vi "Init.vi"(8 "error in (no error)":errorcluster, 10 "PictRef":refnum<vi>, 11 "Menu in":refnum<class "Menu.lvclass">) -> (0 "error out":errorcluster, 2 "MenuSelectionEvent":refnum<user-event>, 3 "Menu out":refnum<class "Menu.lvclass">)   [LabVIEW 2021, in "Menu.lvlib" / "Menu.lvclass"]
uses:
  Menu.lvclass
  MenuSelection.ctl
  Data.ctl
  MenuItems.ctl
  <vilib>/Utility/miscctls.llb/LVMenuShortCut.ctl
  Picture2D/src/Picture/Image.lvclass
  TD_CloseEvent.ctl
  MenuColors.ctl
  Picture2D/src/Color/Color.lvclass
  Picture2D/src/Font/Font.lvclass
  SubMenuIcon.ctl
  Picture2D/src/Picture2D/Picture2D.lvclass
  Menu.lvclass/Menu.ctl
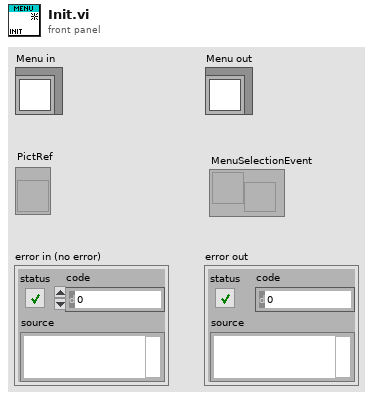
[diagram p1: front panel]
types:
  T1 = typedef "Menu.lvlib/Menu.lvclass/TD_CloseEvent.ctl" = cluster{"Close":bool}
  T2 = typedef "Menu.lvlib/Menu.lvclass/MenuSelection.ctl" = cluster{"ItemTag":string, "ItemPath":string}
  T3 = typedef "Menu.lvlib/Menu.lvclass/Data.ctl" = cluster{"MenuMap":map{string, T4}, "PictRef":refnum<vi>, "MenuSelectionEvent":refnum<user-event>, "TopMenuSpacing":i32, "MenuSpacing":i32, "CloseEvent":refnum<user-event>, "TR_ManageMenuRef":refnum<vi>, "MenuColors":T6, "RTMPath":path, "RTMVIReference":refnum<vi>, "RTMMenuReference":refnum<k9>, "CtlRef":refnum<vi>, "User-Specified Font":refnum<class "Font.lvclass">, "Desired Font":enum16{"User-specified Font", "Application Font", "System Font", "Dialog Font"}, "SubMenuIcon":T7, "SubMenuIconClosed":refnum<class "Picture2D.lvclass">, "SubMenuIconOpened":refnum<class "Picture2D.lvclass">}
  T4 = typedef "Menu.lvlib/Menu.lvclass/MenuItems.ctl" = cluster{"Item Name":string, "Short Cut":T5, "Checked":bool, "Enable":bool, "After item":string, "Item Tags":string[], "Item Names":string[], "Picture":refnum<class "Image.lvclass">, "Hilite Picture":refnum<class "Image.lvclass">, "Displayed":bool}
  T5 = typedef "LVMenuShortCut.ctl" = cluster{"Include Shift Key?":bool, "Include Ctrl Key?":bool, "Shortcut Key":string}
  T6 = typedef "Menu.lvlib/Menu.lvclass/MenuColors.ctl" = cluster{"Text":refnum<class "Color.lvclass">, "HiliteText":refnum<class "Color.lvclass">, "Background":refnum<class "Color.lvclass">, "BorderColor":refnum<class "Color.lvclass">, "Hilite":refnum<class "Color.lvclass">}
  T7 = typedef "Menu.lvlib/Menu.lvclass/SubMenuIcon.ctl" = enum16{"LabVIEW", "Windows", "Custom"}
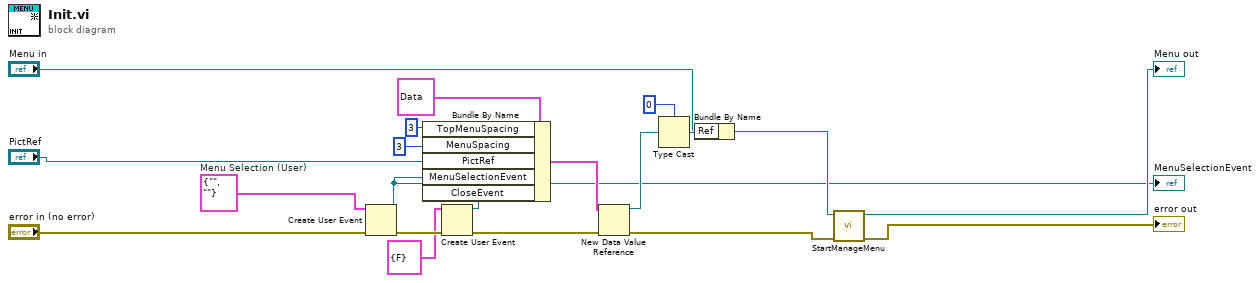
[diagram p0: block diagram]
diagram:
  w5 = T2 {"ItemTag"="", "ItemPath"=""}  # Menu Selection (User)
  n1 = Create User Event(user event datatype=w5, error in="error in (no error)") -> (user event=w2:refnum<user-event>, error out=w13:errorcluster)
  "MenuSelectionEvent" <- w2
  n2 = Create User Event(user event datatype=T1 {"Close"=FALSE} ("CloseEvent"), error in=w13) -> (user event=w10:refnum<user-event>, error out=w12:errorcluster)
  n3 = Bundle By Name(cluster=T3 {"MenuMap"={}, "PictRef"=refnum, "MenuSelectionEvent"=refnum, "TopMenuSpacing"=0, "MenuSpacing"=0, "CloseEvent"=refnum, "TR_ManageMenuRef"=refnum, "MenuColors"={"Text"=refnum, "HiliteText"=refnum, "Background"=refnum, "BorderColor"=refnum, "Hilite"=refnum}, "RTMPath"=path "", "RTMVIReference"=refnum, "RTMMenuReference"=refnum, "CtlRef"=refnum, "User-Specified Font"=refnum, "Desired Font"=enum."User-specified Font", "SubMenuIcon"=enum."LabVIEW", "SubMenuIconClosed"=refnum, "SubMenuIconOpened"=refnum} ("Data"), "TopMenuSpacing"=3, "MenuSpacing"=3, "PictRef"="PictRef", "MenuSelectionEvent"=w2, "CloseEvent"=w10) -> (w16:T3)
  n4 = New Data Value Reference(data value=w16, error in=w12) -> (data value reference=w18:refnum<data-value>, error out=w14:errorcluster)
  n5 = Type Cast(type=u64 0 ("Ref"), x=w18) -> (*(type *) &x=w20:u64)
  n6 = Bundle By Name(cluster="Menu in", "Ref"=w20) -> (w7:refnum<class "Menu.lvclass">)
  n7 = call "StartManageMenu.vi"("error in (no error)"=w14, "Menu in"=w7) -> ("error out"=→"error out":errorcluster, "Menu out"=→"Menu out":refnum<class "Menu.lvclass">)  [unwired: 8 in]
